vi "Main_08A.vi"() -> ()   [LabVIEW 2024]
uses:
  Map_Antena.ctl
  Cluster_Position.ctl
  <vilib>/Utility/miscctls.llb/LVMapReplaceAction.ctl
panel:
  out "Final Grid":string[][](array[string])
  out "Antena Map":T1
  out "Original Grid":string[][](array[string])
  in  "Use Puzzle":bool
  out "Answer 311":u32
  in  "Puzzle":string="............s...............1.....................\n......................E......3.....S..............\n.......................3.....S....................\n...e........T.t.......S.1...........I.............\n..................B..................I.....O......\ng.......z........i39......B..I....................\n.......s....S.......3......................i..I...\n....e.............2..........B....................\n.......tC...z.......g......1......................\n.E......s....R....................................\n..G...t..........2................................\n.........K...C.......2............................\n....T..e...........5...C..........................\n...T................................O...o.........\n...............................g..............o...\n.........z...................g......i............o\n...9.E............H...........Y.......O...........\n..........R..H...............7.O..................\n...........H.............v......7........B........\n..9.Q.......................W......1........Y.....\n.........................z.7.................Y....\n.....Q................................v...........\n....K.......E.....R...............2..........o....\n.n............H......v...........................Y\n.G.y..........................Q...................\n......G....A5.....................h...............\n..........D...5.w...9.............................\n......n....5...L..................................\n............................v.....................\n............L...0t..........7.....................\n..n....k............y....................W........\n..k..........0.........................W..........\n...n.......R..L..a........................W.......\n.........................................h........\n..0..L........c...b...............................\n.....................8.y..........................\n.......w.................6.............h.......N..\n..........y..4....................................\n...0....8...k.....Z........r......................\n..............a...8Z.........G......4.............\n........4..b.q.....................K..............\n.q...........kZ.K......b..D.........d.............\n.8.....................D................r.........\n.....w.........a...............d........A.........\n................................d.A.hV............\n................c..........D.....V....r...........\n.......Z......6.....l........................A.d..\n...................l..6..c....b......r...........N\n......a....4........q..l..V..c................N...\nl.....w...........q..6............V..............."
  in  "Example":string="............\n........0...\n.....0......\n.......0....\n....0.......\n......A.....\n............\n............\n........A...\n.........A..\n............\n............"
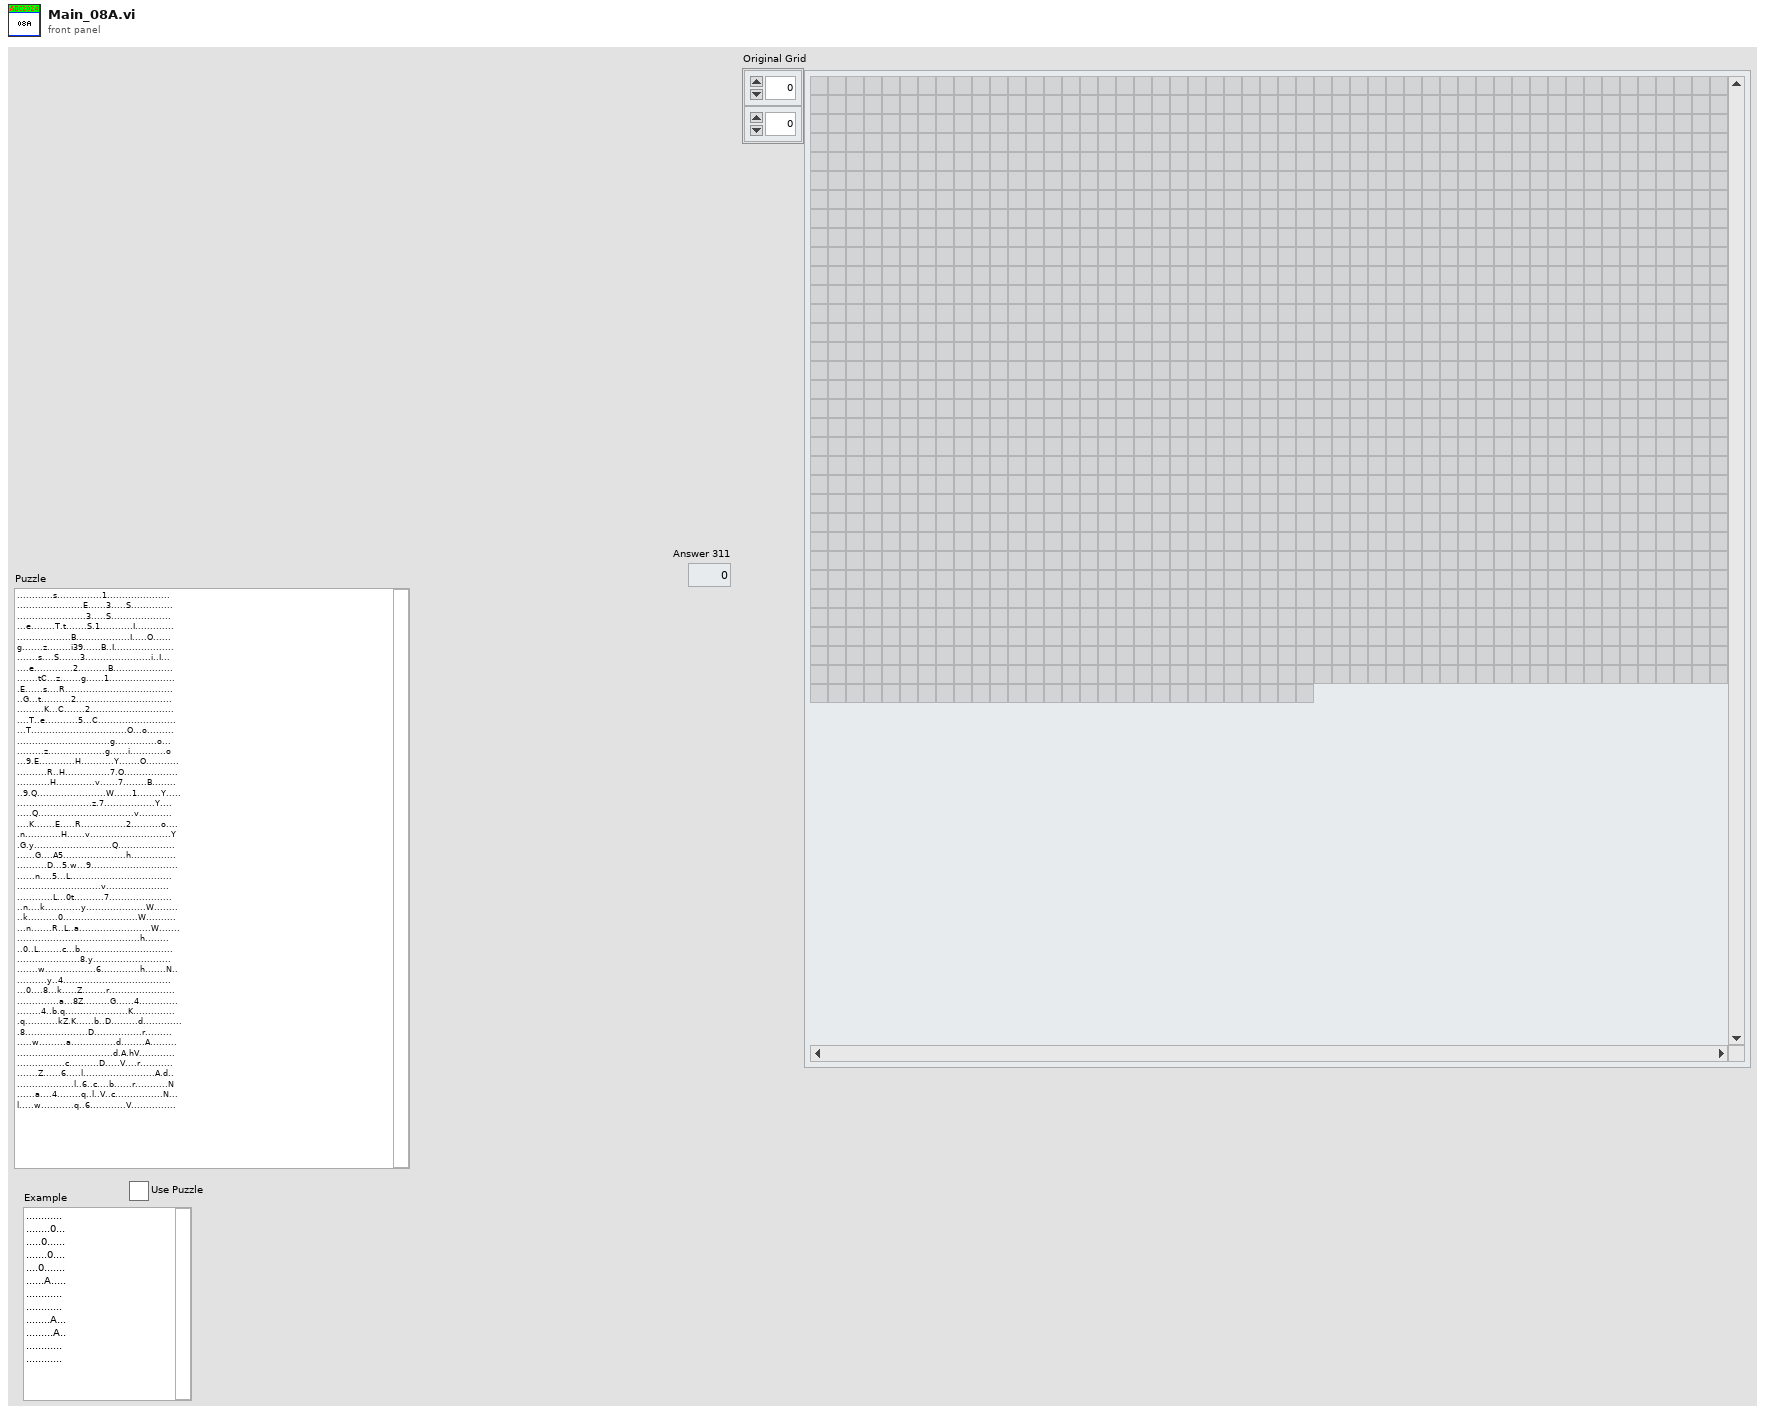
[diagram p1: front panel]
types:
  T1 = typedef "Map_Antena.ctl" = map{string, set{T2}}
  T2 = typedef "Cluster_Position.ctl" = cluster{"R":i32, "C":i32}
  T3 = typedef "LVMapReplaceAction.ctl" = enum32{"Modify Entry only if found", "Add or Modify Entry", "Delete Entry"}
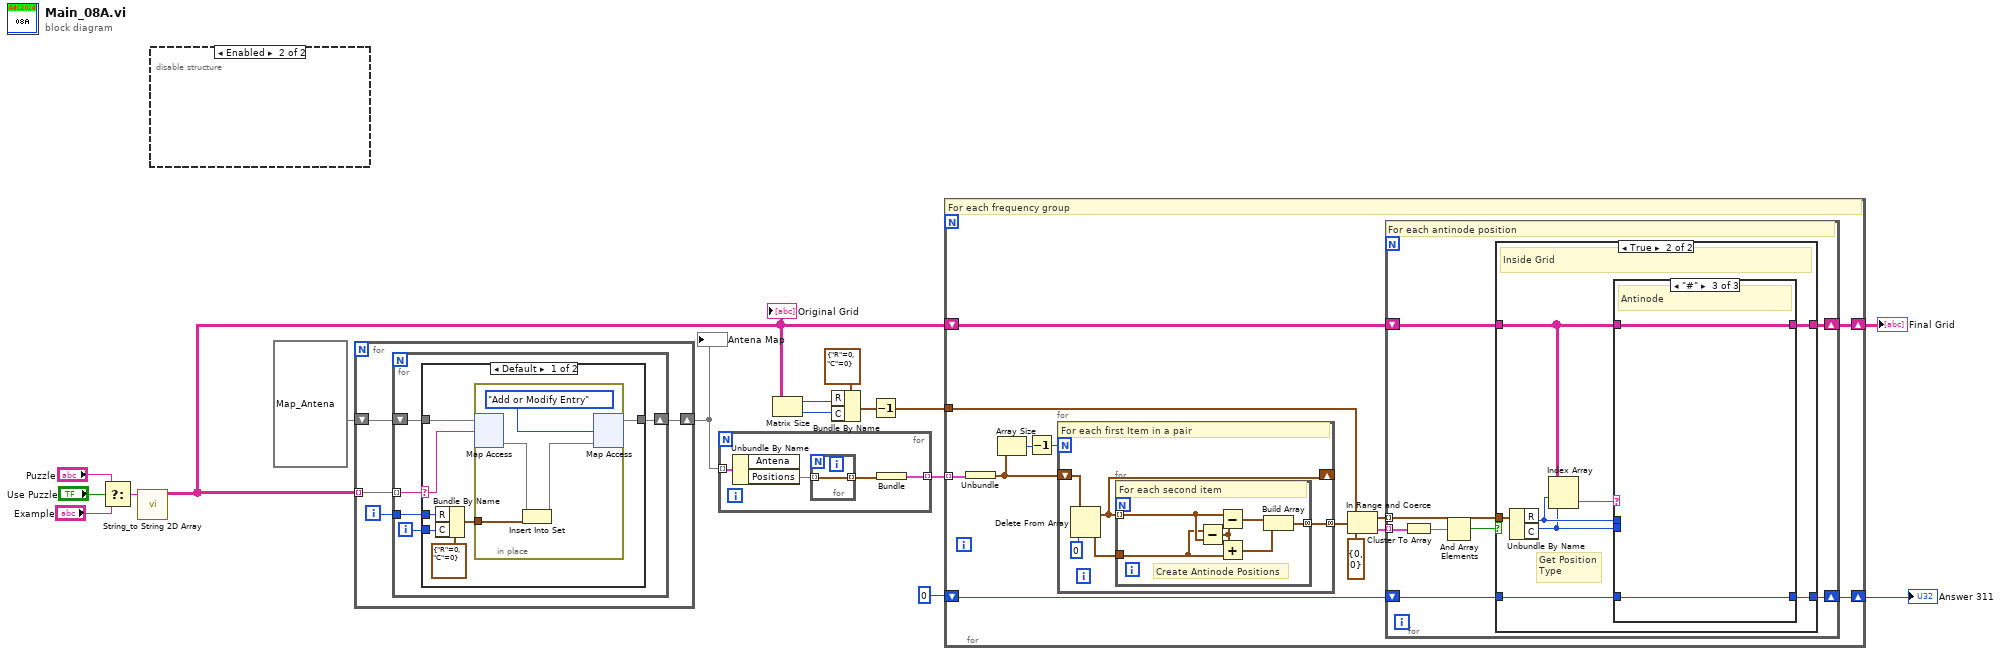
[diagram p0: block diagram]
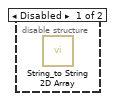
[diagram p3: hidden frame]
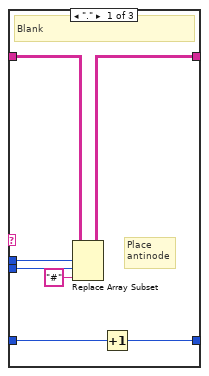
[diagram p5: hidden frame]
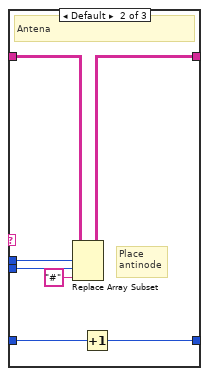
[diagram p6: hidden frame]
diagram:
  n1 = Select(t="Puzzle", s="Use Puzzle", f="Example") -> (s? t:f=w13:string)
  n2 = call "String_to String 2D Array.vi"("Input String"=w13) -> ("2D Array"=w1:string[][])  [unwired: 10 in]
  "Original Grid" <- w1
  n3 = disable-structure shown="Enabled" {
    frame Disabled {
      n4 = call "String_to String 2D Array.vi"() -> ()  [unwired: 11 in, 1 out]
    }
    frame Enabled {
    }
  }
  n5 = for {
    tunnel: w1 -> [w20] mode=indexing
    shift-right: [w18] -> w11
    shift-left: T1 {} ("Antena Map") -> [w19]
    i -> [w17]
    n6 = for {
      tunnel: w20 -> [w25] mode=indexing
      shift-right: [w21] -> w18
      shift-left: w19 -> [w24]
      tunnel: w17 -> [w23]
      i -> [w22]
      n7 = case shown="Default" w25 {
        selector: w25 -> [w31 _]
        tunnel: w24 -> [w32 w37]
        tunnel: w23 -> [w29 _]
        tunnel: w22 -> [w28 _]
        tunnel: [w26 w37] -> w21
        frame Default {
          n8 = Bundle By Name(cluster=T2 {"R"=0, "C"=0} ("Position"), "R"=w29, "C"=w28) -> (w27:T2)
          n9 = in-place {
            in-place-border: w27 -> [w33]
            n10 = in-place-map #1(w32, w31) -> (w35:set{T2})  [unwired: 1 in, 1 out]
            n11 = Insert Into Set(10:w33, 11:w35) -> (3:w34:set{T2})  [unwired: 1 out]
            n12 = in-place-map #1(w34, LVMapReplaceAction."Add or Modify Entry" ("action")) -> (w26:T1)  [unwired: 2 out]
          }
        }
        frame "." {
        }
      }
    }
  }
  "Antena Map" <- w11
  n13 = for {
    tunnel: w11 -> [w41] mode=indexing
    tunnel: [w38] -> w10 mode=indexing
    n14 = Unbundle By Name(w41) -> ("Positions"=w40:set{T2})  [unwired: 1 out]
    n15 = for {
      tunnel: w40 -> [w42] mode=indexing
      tunnel: [w42] -> w39 mode=indexing
    }
    n16 = Bundle(w39) -> (w38:cluster{T2[]})  [unwired: 1 in]
  }
  n17 = Matrix Size(0:w1) -> (1:w8:i32, 2:w7:i32)
  n18 = Bundle By Name(cluster=T2 {"R"=0, "C"=0} ("Position"), "R"=w8, "C"=w7) -> (w6:T2)
  n19 = Decrement(x=w6) -> (x-1=w5:T2)
  n20 = for {
    tunnel: w10 -> [w55] mode=indexing
    tunnel: w5 -> [w50]
    shift-right: [w44] -> w3
    shift-left: u32 0 -> [w45]
    shift-right: [w43] -> w2
    shift-left: w1 -> [w46]
    # "For each frequency group"
    n21 = Unbundle(w55) -> (w54:T2[])
    n22 = Array Size(array=w54) -> (size(s)=w53:i32)
    n23 = Decrement(x=w53) -> (x-1=w52:i32)
    n24 = for {
      N: w52 -> [_]
      shift-right: [w57] -> _
      shift-left: w54 -> [w60]
      tunnel: [w56] -> w51 mode=concatenating
      # "For each first Item in a pair"
      n25 = Delete From Array(array=w60, index=0) -> (deleted portion=w58:T2, array with subset deleted=w57:T2[])  [unwired: 1 in]
      n26 = for {
        tunnel: w58 -> [w63]
        tunnel: w57 -> [w64] mode=indexing
        tunnel: [w66] -> w56 mode=concatenating
        # "Create Antinode Positions"
        # "For each second item"
        n27 = Subtract(x=w63, y=w64) -> (x-y=w65:T2)
        n28 = Subtract(x=w64, y=w65) -> (x-y=w61:T2)
        n29 = Add(x=w65, y=w63) -> (x+y=w62:T2)
        n30 = Build Array(w61, w62) -> (w66:T2[])
      }
    }
    n31 = In Range and Coerce(upper limit=w50, x=w51, lower limit=T2 {"R"=0, "C"=0}) -> (coerced(x)=w47:T2[], In Range?=w48:cluster{"R":bool, "C":bool}[])
    n32 = for {
      tunnel: w48 -> [w74] mode=indexing
      tunnel: w47 -> [w71] mode=indexing
      shift-right: [w69] -> w43
      shift-left: w46 -> [w70]
      shift-right: [w67] -> w44
      shift-left: w45 -> [w68]
      # "For each antinode position"
      n33 = Cluster To Array(cluster=w74) -> (array=w73:bool[])
      n34 = And Array Elements(Boolean array=w73) -> (logical AND=w72:bool)
      n35 = case shown="True" w72 {
        tunnel: w71 -> [_ w82]
        tunnel: w70 -> [w76 w83]
        tunnel: [w76 w79] -> w69
        tunnel: w68 -> [w75 w78]
        tunnel: [w75 w77] -> w67
        frame False {
          # "Off Grid"
        }
        frame True {
          # "Get Position\nType"
          # "Inside Grid"
          n36 = Unbundle By Name(w82) -> ("R"=w81:i32, "C"=w80:i32)
          n37 = Index Array(array=w83, index (row)=w81, index (col)=w80) -> (element=w84:string)
          n38 = case shown="\"#\"" w84 {
            tunnel: w83 -> [w91 w98 w100]
            tunnel: w81 -> [w89 w96 _]
            tunnel: w80 -> [w88 w95 _]
            tunnel: [w90 w97 w100] -> w79
            tunnel: w78 -> [w86 w93 w99]
            tunnel: [w85 w92 w99] -> w77
            frame "." {
              # "Place\nantinode"
              # "Blank"
              n39 = Replace Array Subset(array=w91, new element="#" ("new element/subarray"), index (row)=w89, index (col)=w88) -> (w90:string[][])
              n40 = Increment(x=w86) -> (x+1=w85:u32)
            }
            frame Default {
              # "Place\nantinode"
              # "Antena"
              n41 = Replace Array Subset(array=w98, new element="#" ("new element/subarray"), index (row)=w96, index (col)=w95) -> (w97:string[][])
              n42 = Increment(x=w93) -> (x+1=w92:u32)
            }
            frame "#" {
              # "Antinode"
            }
          }
        }
      }
    }
  }
  "Answer 311" <- w3
  "Final Grid" <- w2
